vi "dP_data_labels.vi"() -> (0 "dP Data Labels":string[](array[string])=["Timestamp", "Vap Mass Flow", "Liq Mass Flow", "DP", "Liq Tank P", "LiqTank T", "Sep P", "SepT", "Liq In P", "Liq In T", "Vap Tank P", "Vap Tank T", "Dev Section P", "Dev Section T", "Up TS P", "Up TS T", "Low TS P", "Low TS T", "Cond Top T", "Evap Top T", "Cond Bot T", "Evap Bot T", "Win 3-4 P", "Top Heat T", "Bot Heat T", ""])   [LabVIEW 2015]
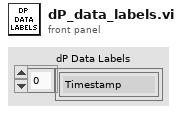
[diagram p1: front panel]
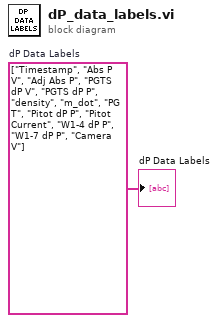
[diagram p0: block diagram]
diagram:
  w1 = string[] ["Timestamp", "Abs P V", "Adj Abs P", "PGTS dP V", "PGTS dP P", "density", "m_dot", "PG T", "Pitot dP P", "Pitot Current", "W1-4 dP P", "W1-7 dP P", "Camera V"]  # dP Data Labels
  "dP Data Labels" <- w1
